vi "Do Main Action.vi"(8 "error in (no error)":errorcluster, 10 "AbstractData":refnum<class "AbstractData.lvclass">, 11 "ReadoutDevice in":refnum<class "ReadoutDevice.lvclass">) -> (0 "error out":errorcluster, 3 "ReadoutDevice out":refnum<class "ReadoutDevice.lvclass">)   [LabVIEW 2014, in "ReadoutDevice.lvclass"]
uses:
  ReadoutDevice.lvclass
  Model/Data/AbstractData/AbstractData.lvclass
  <vilib>/ActorFramework/Message Enqueuer/Init from Existing Queue.vi
  <vilib>/ActorFramework/Message Enqueuer/Enqueue.vi
  <vilib>/ActorFramework/Message Priority Queue/Priority Enqueue.vi
  <vilib>/ActorFramework/Message Enqueuer/Message Priority.ctl
  <vilib>/ActorFramework/Message Enqueuer/Message Enqueuer.lvclass
  Interfaces/Pipelined Actor/Pipelined Actor Messages/Do Main Action Msg/Do Main Action Msg.lvclass
  Device/Device.lvclass
  <vilib>/ActorFramework/Actor/Actor.lvclass
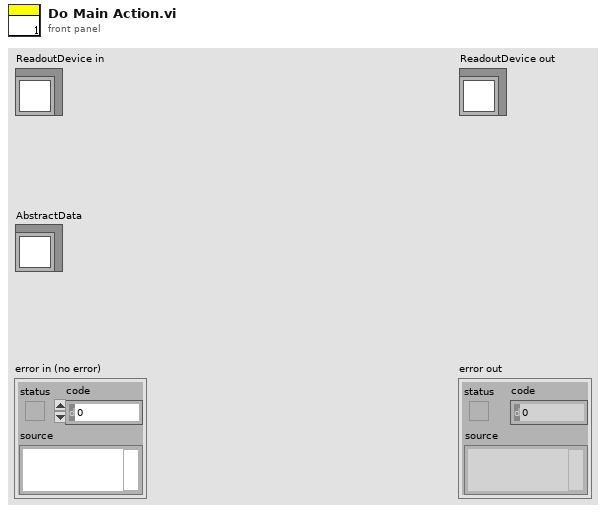
[diagram p1: front panel]
types:
  T1 = typedef "Actor Framework.lvlib/Message Enqueuer.lvclass/Message Priority.ctl" = enum16{"Low", "Normal", "High"}
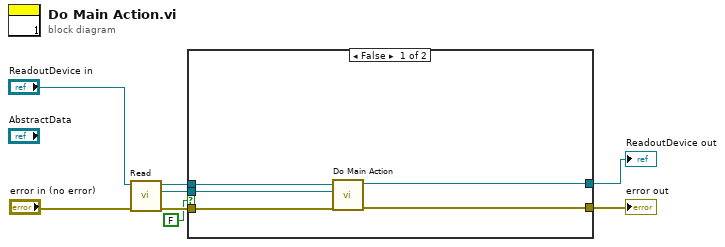
[diagram p0: block diagram]
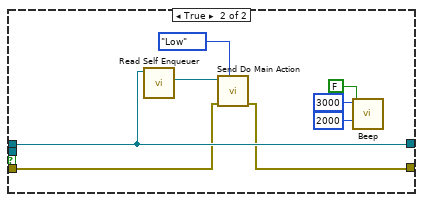
[diagram p2: hidden frame]
diagram:
  n1 = call-dynamic "Read.vi"("error in (no error)"="error in (no error)", "ReadoutDevice in"="ReadoutDevice in") -> ("error out"=w3:errorcluster, "Data"=w5:refnum<class "AbstractData.lvclass">, "ReadoutDevice out"=w6:refnum<class "ReadoutDevice.lvclass">)  [unwired: 6 in, 1 out]
  n2 = case shown="False" FALSE {
    tunnel: [w13 w18] -> w8
    tunnel: [w12 w21] -> w7
    tunnel: w6 -> [w11 w21]
    tunnel: w5 -> [w9 _]
    tunnel: w3 -> [w10 w19]
    frame False {
      n3 = call-parent "Do Main Action.vi"("error in (no error)"=w10, "AbstractData"=w9, "Pipelined Actor in"=w11) -> ("error out"=w13:errorcluster, "Pipelined Actor out"=w12:refnum<class "ReadoutDevice.lvclass">)  [unwired: 7 in]
    }
    frame True {
      n4 = call <vilib>:"Read Self Enqueuer.vi"("Actor"=w21) -> ("Self Enqueuer"=w20:refnum<class "Message Enqueuer.lvclass">)  [unwired: 10 in]
      n5 = call "Send Do Main Action.vi"("Message Priority (Normal)"=Message_Priority."Low", "error in (no error)"=w19, "Message Enqueuer"=w20) -> ("error out"=w18:errorcluster)  [unwired: 7 in, 1 out]
      n6 = call <vilib>:"Beep.vi"("use system alert? (T)"=FALSE, "duration (msec)"=u32 2000, "frequency (Hz)"=u32 3000) -> ()  [unwired: 9 in]
    }
  }
  "error out" <- w8
  "ReadoutDevice out" <- w7
